vi "OpenCamera.vi"(8 "error in (no error)":errorcluster, 10 "Camera Occurance":refnum<k4>) -> (0 "error out":errorcluster, 3 "SerialRefOut":T1)   [LabVIEW 2017, in "VisionHW.lvlib"]
uses:
  VisionHW.lvlib
  <vilib>/Rock Robotics/WPI/SerialPort/WPI_SerialPortRef.ctl
  <vilib>/Rock Robotics/WPI/SerialPort/WPI_SerialPort.ctl
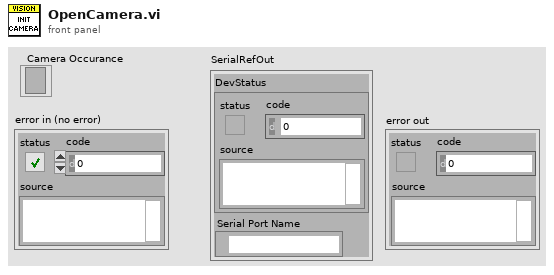
[diagram p1: front panel]
types:
  T1 = typedef "WPI_SerialPortRef.ctl" = cluster{"DevStatus":errorcluster, "Serial Port Name":refnum<visa-resource-name>}
  T2 = typedef "WPI_SerialPort.ctl" = enum16{"Onboard RS-232", "MXP TTL", "USB 1", "USB 2"}
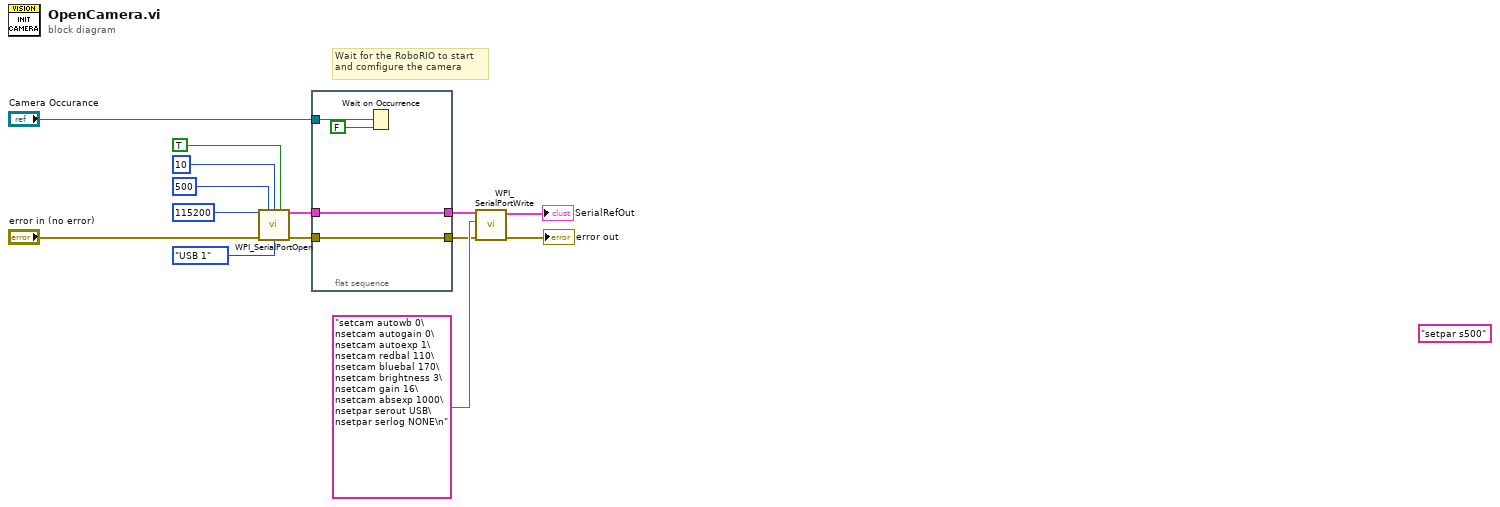
[diagram p0: block diagram]
diagram:
  (unwired) "setpar s500" ("write buffer")
  # "Wait for the RoboRIO to start\nand comfigure the camera"
  n1 = call <vilib>:"WPI_SerialPortOpen.vi"("Baud Rate"=u32 115200, "Timeout Value (ms)"=u32 500, "Termination Char (0xA = '\\n' = LF)"=u8 10 ("Termination Char (0xA = '\\n' = LF)"), "Enable Termination Char? (T)"=TRUE, "error in (no error)"="error in (no error)", "Serial Port"=WPI_SerialPort."USB 1") -> ("SerialPortRef"=w5:T1, "error out"=w4:errorcluster)  [unwired: 8 in]
  n2 = flat-sequence {
    tunnel: w5 -> [w17]
    tunnel: w4 -> [w18]
    tunnel: [w17] -> w3
    tunnel: [w18] -> w2
    tunnel: "Camera Occurance" -> [w16]
    frame #0 {
      n3 = Wait on Occurrence(1:FALSE ("ignore previous (T)"), 2:w16) -> ()  [unwired: 1 in, 1 out]
    }
  }
  n4 = call <vilib>:"WPI_SerialPortWrite.vi"("error in (no error)"=w2, "Buffer"="setcam autowb 0\nsetcam autogain 0\nsetcam autoexp 1\nsetcam redbal 110\nsetcam bluebal 170\nsetcam brightness 3\nsetcam gain 16\nsetcam absexp 1000\nsetpar serout USB\nsetpar serlog NONE\n" ("write buffer"), "SerialPortRef"=w3) -> ("error out"=→"error out":errorcluster, "SerialPortRef"=→"SerialRefOut":T1)  [unwired: 6 in, 1 out]
